vi "_Read (No Objects).vi"(8 "error in (no error)":errorcluster, 11 "Cluster In":T10={"Channel Names"=[], "Channel Units"=[], "Most Recent Data Points"=[], "History Buffers"=[], "Ring Buffers"=[], "Exp Range Min"=0, "Exp Range Max"=0, "exposure mode"=enum."manual", "operation (meas. mode)"=enum."Measurement mode", "Exposure (ms)"=0, "Quiet Errors?"=FALSE, "Error Status"={"status"=FALSE, "code"=0, "source"=""}}) -> (0 "error out":errorcluster, 2 "4 Data Points":dbl[](array[numeric]), 3 "Cluster Out":T10={"Channel Names"=[], "Channel Units"=[], "Most Recent Data Points"=[], "History Buffers"=[], "Ring Buffers"=[], "Exp Range Min"=0, "Exp Range Max"=0, "exposure mode"=enum."manual", "operation (meas. mode)"=enum."Measurement mode", "Exposure (ms)"=0, "Quiet Errors?"=FALSE, "Error Status"={"status"=FALSE, "code"=0, "source"=""}})   [LabVIEW 2009]
uses:
  Utility Classes/Readable/Channel Names.ctl
  Utility Classes/Readable/Channel Units.ctl
  Utility Classes/Readable/Data Points.ctl
  Utility Classes/Readable/Data Point.ctl
  Utility Classes/Readable/Time.ctl
  Utility Classes/Readable/X.ctl
  Utility Classes/Readable/TX Graph.ctl
  HighFinesse WS5/Variable Typedefs.llb/Exposure Mode.ctl
  HighFinesse WS5/Control typedefs.llb/Measurement Mode.ctl
  HighFinesse WS5/HighFinesse WS5.lvlib
  Utility Classes/Readable/Readable.lvclass
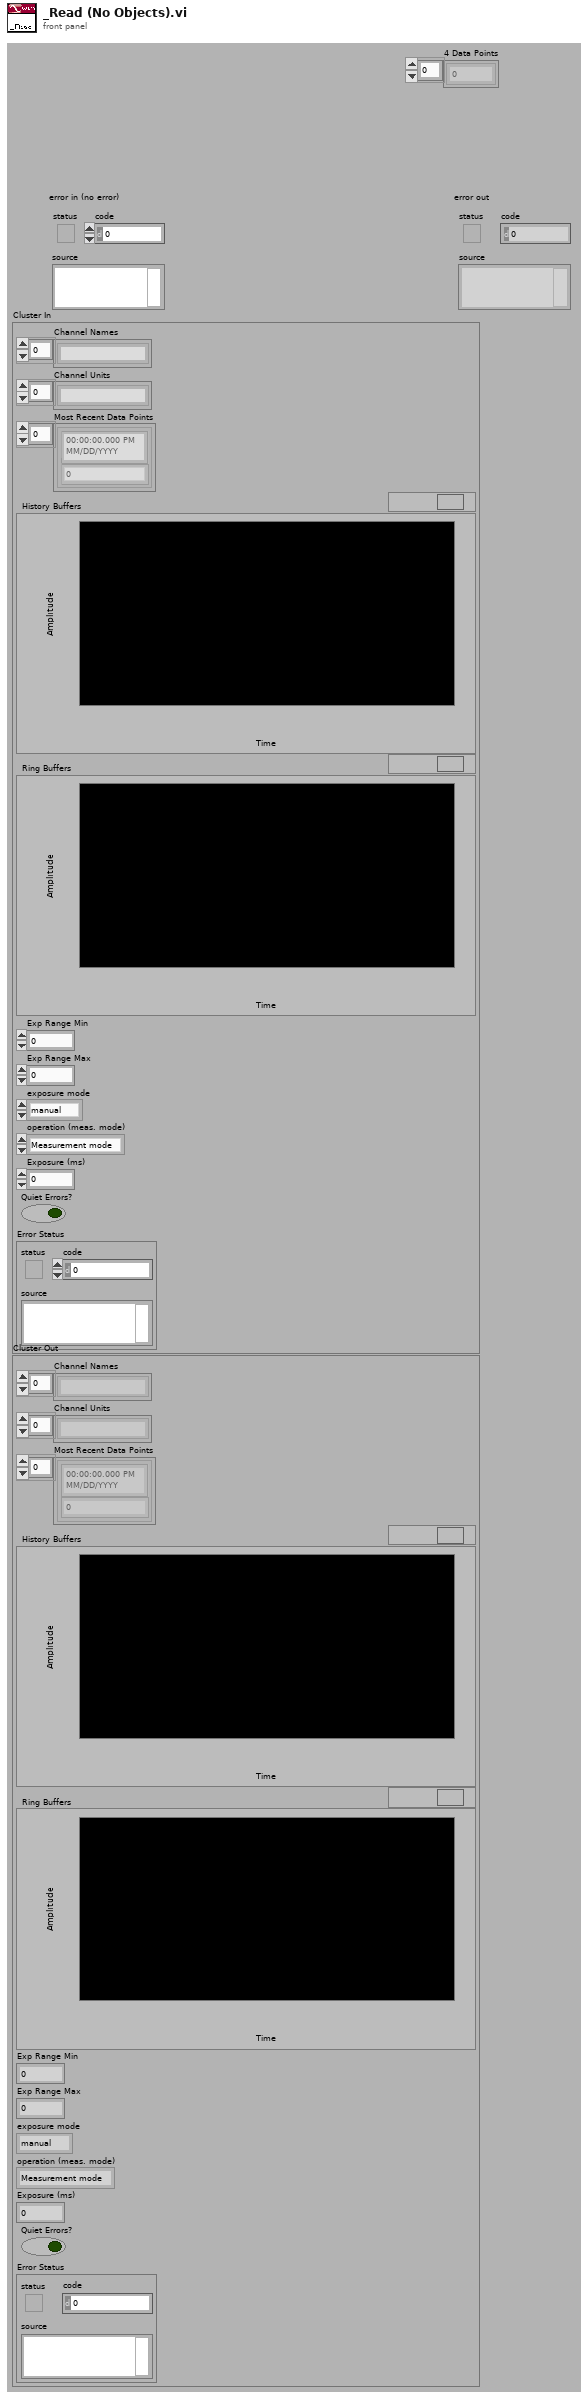
[diagram p1: front panel]
types:
  T1 = typedef "Readable.lvclass/Channel Names.ctl" = string[]
  T2 = typedef "Readable.lvclass/Channel Units.ctl" = string[]
  T3 = typedef "Readable.lvclass/Data Points.ctl" = T4[]
  T4 = typedef "Readable.lvclass/Data Point.ctl" = cluster{"t":T5, "x":T6}
  T5 = typedef "Readable.lvclass/Time.ctl" = timestamp
  T6 = typedef "Readable.lvclass/X.ctl" = dbl
  T7 = typedef "Readable.lvclass/TX Graph.ctl" = cluster{"Data Points":cluster{"t":timestamp, "x":dbl}[]}[]
  T8 = typedef "HighFinesse WS5.lvlib/Exposure Mode.ctl" = enum16{"manual", "automatic"}
  T9 = typedef "HighFinesse WS5.lvlib/Measurement Mode.ctl" = enum16{"Measurement off", "Adjustment mode", "Measurement mode"}
  T10 = cluster{"Channel Names":T1, "Channel Units":T2, "Most Recent Data Points":T3, "History Buffers":T7, "Ring Buffers":T7, "Exp Range Min":u32, "Exp Range Max":u32, "exposure mode":T8, "operation (meas. mode)":T9, "Exposure (ms)":u16, "Quiet Errors?":bool, "Error Status":errorcluster}
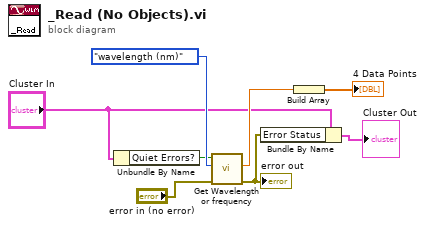
[diagram p0: block diagram]
diagram:
  n1 = Unbundle By Name("Cluster In") -> ("Quiet Errors?"=w5:bool)
  n2 = call "Get Wavelength or frequency.vi"("error in (no error)"="error in (no error)", "mode (wavelength)"=enum16{"wavelength (nm)", "frequency (THz)"}."wavelength (nm)", "Quiet Errors?"=w5) -> ("error out"=w4:errorcluster, "result"=w7:dbl)  [unwired: 1 in, 6 out]
  "error out" <- w4
  n3 = Bundle By Name(cluster="Cluster In", "Error Status"=w4) -> (→"Cluster Out":T10)
  n4 = Build Array(w7) -> (→"4 Data Points":dbl[])
